vi "Generate Headers.vi"(10 "Content Body (Empty)":string, 11 "Client Data":T1) -> (2 "x-ni-date":string, 3 "x-ni-authentication":string)   [LabVIEW 2020, in "WS Admin.lvlib"]
uses:
  WS Admin.lvlib
  Client Data.ctl
  HTTP Method.ctl
  <vilib>/IlluminatedG/lv-web-crypto/lv-crypto/Crypto/Hashes/MD5/MD5.lvclass
  <vilib>/IlluminatedG/lv-web-crypto/lv-crypto/Crypto/Hashes/SHA-256/SHA-256.lvclass
  <vilib>/IlluminatedG/lv-web-crypto/lv-crypto/Crypto/Crypto.lvlib
  <vilib>/IlluminatedG/lv-web-crypto/lv-base64/Base64.lvlib
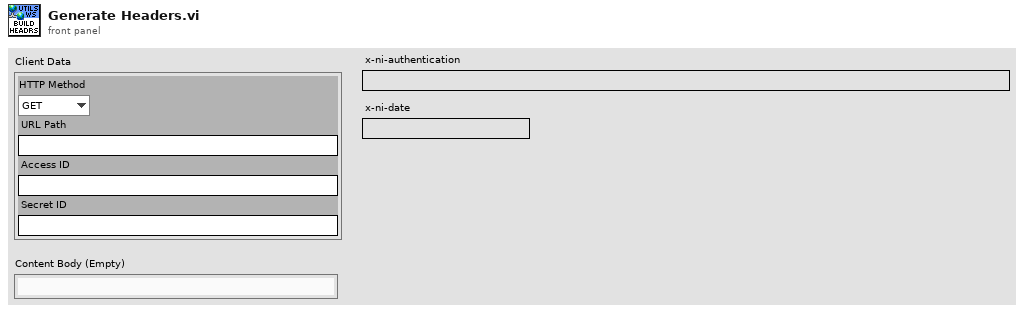
[diagram p1: front panel]
types:
  T1 = typedef "WS Admin.lvlib/Client Data.ctl" = cluster{"HTTP Method":T2, "URL Path":string, "Access ID":string, "Secret ID":string}
  T2 = typedef "WS Admin.lvlib/HTTP Method.ctl" = enum16{"GET", "POST", "PUT", "DELETE"}
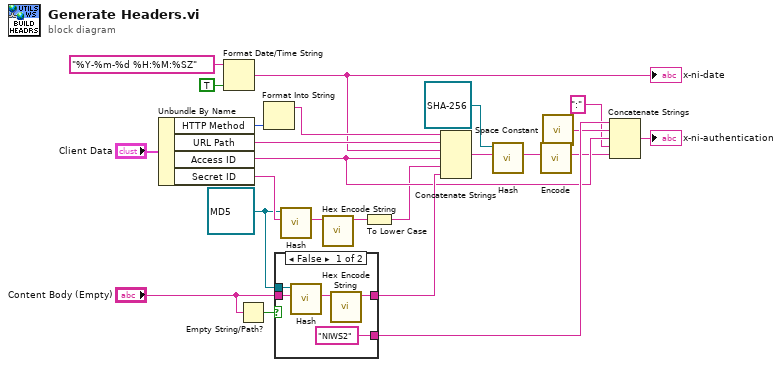
[diagram p0: block diagram]
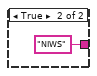
[diagram p2: hidden frame]
diagram:
  w15 = refnum<class "MD5.lvclass"> refnum ("Crypto.lvlib:MD5.lvclass")
  n1 = Unbundle By Name("Client Data") -> ("HTTP Method"=w21:T2, "URL Path"=w20:string, "Access ID"=w6:string, "Secret ID"=w18:string)
  n2 = Format Date/Time String(time format string (%c)="%Y-%m-%d %H:%M:%SZ", UTC format=TRUE) -> (date/time string=w1:string)  [unwired: 1 in]
  "x-ni-date" <- w1
  n3 = Empty String/Path?(string/path="Content Body (Empty)") -> (empty?=w13:bool)
  n4 = Format Into String(w21) -> (resulting string=w19:string)  [unwired: 3 in, 1 out]
  n5 = case shown="False" w13 {
    tunnel: w15 -> [w28 _]
    tunnel: "Content Body (Empty)" -> [w27 _]
    tunnel: [w26 _] -> w12
    tunnel: ["NIWS2" "NIWS"] -> w8
    frame False {
      n6 = call-dynamic "Hash.vi"("Message"=w27, "MD5 in"=w28) -> ("Hash"=w29:string)  [unwired: 7 in, 2 out]
      n7 = call <vilib>:"Hex Encode String.vi"("String"=w29) -> ("Hex Encoded String"=w26:string)  [unwired: 10 in]
    }
    frame True {
    }
  }
  n8 = call-dynamic "Hash.vi"("Message"=w18, "MD5 in"=w15) -> ("Hash"=w17:string)  [unwired: 7 in, 2 out]
  n9 = call <vilib>:"Hex Encode String.vi"("String"=w17) -> ("Hex Encoded String"=w16:string)  [unwired: 10 in]
  n10 = To Lower Case(string=w16) -> (all lower case string=w2:string)
  n11 = Concatenate Strings(w19, w20, w1, w6, w2, w12) -> (w10:string)
  n12 = call-dynamic "Hash.vi"("Message"=w10, "SHA-256 in"=refnum<class "SHA-256.lvclass"> refnum ("Crypto.lvlib:SHA-256.lvclass")) -> ("Hash"=w9:string)  [unwired: 7 in, 2 out]
  n13 = call <vilib>:"Encode.vi"("string in (not encoded)"=w9) -> ("string out (base64-encoded)"=w5:string)  [unwired: 9 in, 1 out]
  n14 = call <vilib>:"Space Constant.vi"() -> ("String"=w7:string)
  n15 = Concatenate Strings(w8, w7, w6, ":", w5) -> (→"x-ni-authentication":string)
